vi "Request Synchronous Data (Variant).vi"(6 "Ignore Past Updates? (F)":bool, 7 "Timeout In ms (-1)":i32=-1, 8 "error in (no error)":errorcluster, 9 "Type":variant, 10 "Datum Name":string, 11 "IModel In":refnum<class "IModel.lvclass">) -> (0 "error out":errorcluster, 1 "timed out?":bool, 2 "Data":variant, 4 "Publication Time":timestamp)   [LabVIEW 2017, in "IModel.lvlib" / "IModel.lvclass"]
doc: "DEPRECATED by IObserver.lvclass: Request Synchronous Data.vim"
uses:
  IModel.lvclass
  C:/Git/mva-framework/Source/Framework/IObserver/IObserver/IObserver.lvclass
  IObserver/IObserver/IObserver.lvclass/IObserver.ctl
  SubscriptionPolicy/OneShotSubscription/OneShotSubscription.lvclass/OneShotSubscription.ctl
  gpm_packages/@cs/transport/Source/Concrete/NotifierTransport/NotifierTransport.lvclass/NotifierTransport.ctl
  IMediator/SubscriptionRequest/SubscriptionRequest.lvclass/SubscriptionRequest.ctl
  AbstractMessages/PreAddressedMsg/PreAddressedMsg.lvclass/PreAddressedMsg.ctl
  IMediator/IMediator Messages/Subscribe Msg/Subscribe Msg.lvclass/Subscribe Msg.ctl
  <vilib>/ActorFramework/Message Enqueuer/Message Enqueuer.lvclass/Message Enqueuer.ctl
  <vilib>/ActorFramework/Message Enqueuer/Enqueue.vi
  AbstractMessages/PreAddressedMsg/Read Return Address.vi
  gpm_packages/@cs/transport/Source/Concrete/NotifierTransport/NotifierTransport.lvclass
  C:/Git/mva-framework/gpm_packages/@cs/transport/Source/ITransport/ITransport.lvclass
  SubscriptionPolicy/OneShotSubscription/OneShotSubscription.lvclass
  C:/Git/mva-framework/Source/Framework/IMediator/ISubscriptionPolicy/ISubscriptionPolicy.lvclass
  IMediator/IMediator Messages/Subscribe Msg/Subscribe Msg.lvclass
  C:/Git/mva-framework/Source/Framework/AbstractMessages/PreAddressedMsg/PreAddressedMsg.lvclass
  C:/Program Files (x86)/National Instruments/LabVIEW 2017/vi.lib/ActorFramework/Message/Message.lvclass
  <vilib>/Utility/error.llb/Error Cluster From Error Code.vi
  <vilib>/ActorFramework/Message Priority Queue/Priority Enqueue.vi
  IMediator/SubscriptionRequest/SubscriptionRequest.lvclass
  IMediator/ISubscriptionPolicy/ISubscriptionPolicy.lvclass
  IObserver/IObserver/IObserver.lvclass
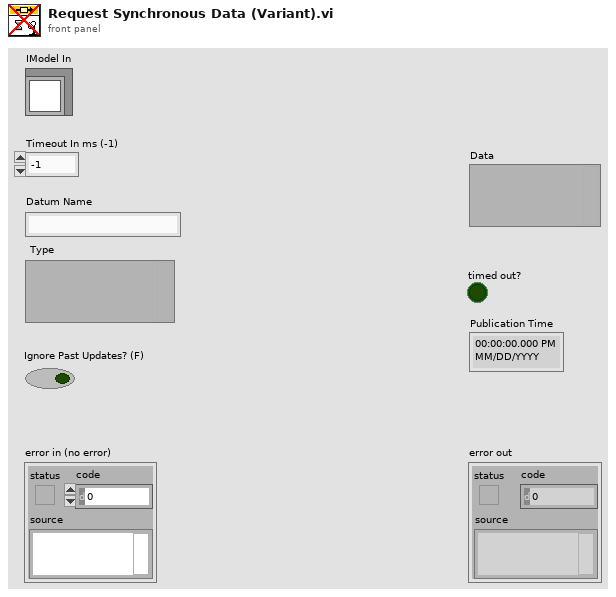
[diagram p1: front panel]
types:
  T1 = typedef "IMediator.lvlib/ISubscriptionPolicy.lvclass/ISubscriptionPolicy Reference.ctl" = refnum<data-value>
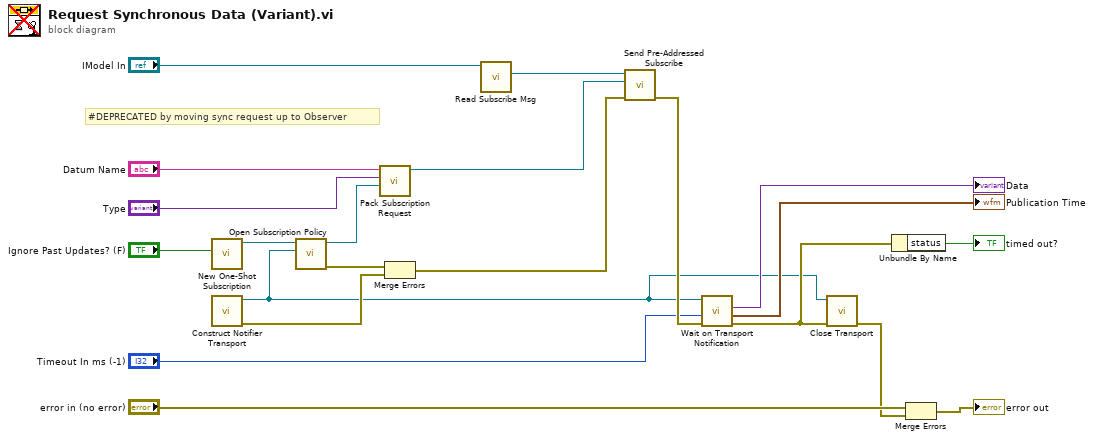
[diagram p0: block diagram]
diagram:
  # "#DEPRECATED by moving sync request up to Observer"
  n1 = call "New One-Shot Subscription.vi"("Ignore Past Updates? (F)"="Ignore Past Updates? (F)") -> ("OneShotSubscription Out"=w18:refnum<class "OneShotSubscription.lvclass">)  [unwired: 10 in]
  n2 = call "Construct Notifier Transport.vi"() -> ("error out"=w12:errorcluster, "NotifierTransport"=w1:refnum<class "NotifierTransport.lvclass">)  [unwired: 10 in]
  n3 = call "Open Subscription Policy.vi"("Transport"=w1, "SubscriptionPolicy"=w18) -> ("error out"=w14:errorcluster, "Subscription Policy"=w3:T1)  [unwired: 8 in]
  n4 = call "Pack Subscription Request.vi"("Subscription Policy"=w3, "Type"="Type", "Datum Name"="Datum Name") -> ("SubscriptionRequest"=w15:refnum<class "SubscriptionRequest.lvclass">)  [unwired: 8 in]
  n5 = Merge Errors(w14, w12) -> (w13:errorcluster)
  n6 = call "Read Subscribe Msg.vi"("IObserver in"="IModel In") -> ("Pre-Addressed Subscribe Msg"=w16:refnum<class "Subscribe Msg.lvclass">)  [unwired: 10 in]
  n7 = call "Send Pre-Addressed Subscribe.vi"("error in (no error)"=w13, "Subscription Request"=w15, "Subscribe Msg"=w16) -> ("error out"=w11:errorcluster)  [unwired: 8 in]
  n8 = call "Wait on Transport Notification.vi"("error in (no error)"=w11, "Timeout In ms (-1)"="Timeout In ms (-1)", "NotifierTransport"=w1) -> ("error out"=w4:errorcluster, "Publication Time"=→"Publication Time":timestamp, "Data"=→"Data":variant)  [unwired: 6 in]
  n9 = call-dynamic "Close Transport.vi"("error in (no error)"=w4, "NotifierTransport"=w1) -> ("error out"=w6:errorcluster)  [unwired: 9 in]
  n10 = Unbundle By Name(w4) -> ("status"=→"timed out?":bool)
  n11 = Merge Errors("error in (no error)", w6) -> (→"error out":errorcluster)
